vi "Main.vi"(8 "error in (no error)":T2) -> (0 "error out":T2)   [LabVIEW 2019, in "DataManagment.lvlib"]
doc: "Manages burst data\n\nHandles tx bursts \"library\", collects rx bursts for later retrieving.\nManages bursts in memory and on drive"
uses:
  DataManagment.lvlib
  DM group info.ctl
  module data.ctl
  SubVIs/mmWave data_class/mmWave data.lvclass
  DM signal group.ctl
  Intertarget communication/Command + data + response cluster.ctl
  Intertarget communication/Status + response + data cluster.ctl
  module state.ctl
  DM get burst parameters.ctl
  DM get burst by index parameters.ctl
  5bf6cc24-2521-4779-a80f-885c0f377251.vi
  171e3bb6-d49a-4f23-9fbb-f47b30baaa7f.vi
  a598079f-c5bd-4db8-828d-75a2daebc4d7.vi
  ee899b51-2d5d-4f26-9c2b-9d2f7332cf3c.vi
  697aacd5-9936-4587-9d14-828a3325ba78.vi
  6dd8da64-2a06-40fc-b69d-37d6f9184272.vi
  171e3bb6-d49a-4f23-9fbb-f47b30baaa7f.vi/5cbf4985-03a2-482f-aa1d-412015602fcf.vi
  171e3bb6-d49a-4f23-9fbb-f47b30baaa7f.vi/9ddd5499-773d-48fa-be3a-3edd2f81d7af.vi
  a598079f-c5bd-4db8-828d-75a2daebc4d7.vi/43a70c26-45ca-4555-8713-4d640d2761cd.vi
  a598079f-c5bd-4db8-828d-75a2daebc4d7.vi/532e6f42-99be-4d49-9f37-ebc30de797f6.vi
  ee899b51-2d5d-4f26-9c2b-9d2f7332cf3c.vi/279be3f1-d035-438d-8d75-920168a460ff.vi
  ee899b51-2d5d-4f26-9c2b-9d2f7332cf3c.vi/125f3e28-a4cf-4289-b3e7-931c39c491a6.vi
  697aacd5-9936-4587-9d14-828a3325ba78.vi/bc4ebb1e-c054-43e7-8435-a2cc996418b2.vi
  697aacd5-9936-4587-9d14-828a3325ba78.vi/c68d463f-3934-40a4-88c5-9e6f02909ca2.vi
  6dd8da64-2a06-40fc-b69d-37d6f9184272.vi/4dacbd5d-4013-4b6b-9f66-fc6ac213e238.vi
  6dd8da64-2a06-40fc-b69d-37d6f9184272.vi/8eb97bab-6edf-4927-bcd5-73d21db452ab.vi
  <vilib>/Utility/High Resolution Relative Seconds.vi
  DM GV.vi
  SubVIs/Shared/Comm GV.vi
  <vilib>/addons/_JKI.lib/Serialization/JSON/Library/Unflatten From JSON String.vi
  Intertarget communication/CommandResponse communication.lvlib
  SubVIs/Shared/Shared.lvlib
  <vilib>/addons/_JKI.lib/Serialization/JSON/JKI JSON Serialization.lvlib
panel:
  out "group info":T1 {"Memory" format="%#_6pB"; "burst sizes" format="%#_6p"}
  out "oldest":string
  out "newest":string
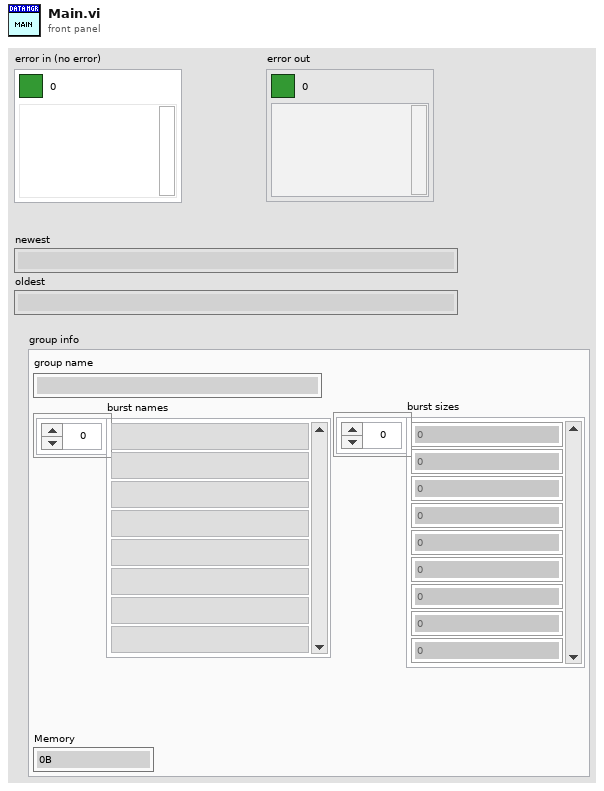
[diagram p1: front panel]
types:
  T1 = typedef "DataManagment.lvlib/DM group info.ctl" = cluster{"group name":string, "burst names":string[], "burst sizes":dbl[], "Memory":dbl}
  T2 = cluster{"Boolean Round":bool, "code":i32, "source":string}
  T3 = typedef "CommandResponse communication.lvlib/Command + data + response cluster.ctl" = cluster{"message":string, "parameters":string, "response notifier":refnum<notifier>, "data":variant}
  T4 = typedef "DataManagment.lvlib/module state.ctl" = enum16{"init", "configure", "run", "close"}
  T5 = typedef "DataManagment.lvlib/module data.ctl" = cluster{"Group names":string[], "Signal groups":map{string, refnum<class "mmWave data.lvclass">}[], "groups":T6[]}
  T6 = typedef "DataManagment.lvlib/DM signal group.ctl" = cluster{"history":string[]}
  T7 = typedef "CommandResponse communication.lvlib/Status + response + data cluster.ctl" = cluster{"message":string, "response":string, "data":variant}
  T8 = typedef "DataManagment.lvlib/DM get burst parameters.ctl" = cluster{"group":string, "bursts":string[]}
  T9 = typedef "DataManagment.lvlib/DM get burst by index parameters.ctl" = cluster{"group":string, "index":i32}
  T10 = map{string, refnum<class "mmWave data.lvclass">}[]
  T11 = cluster{string, refnum<class "mmWave data.lvclass">}
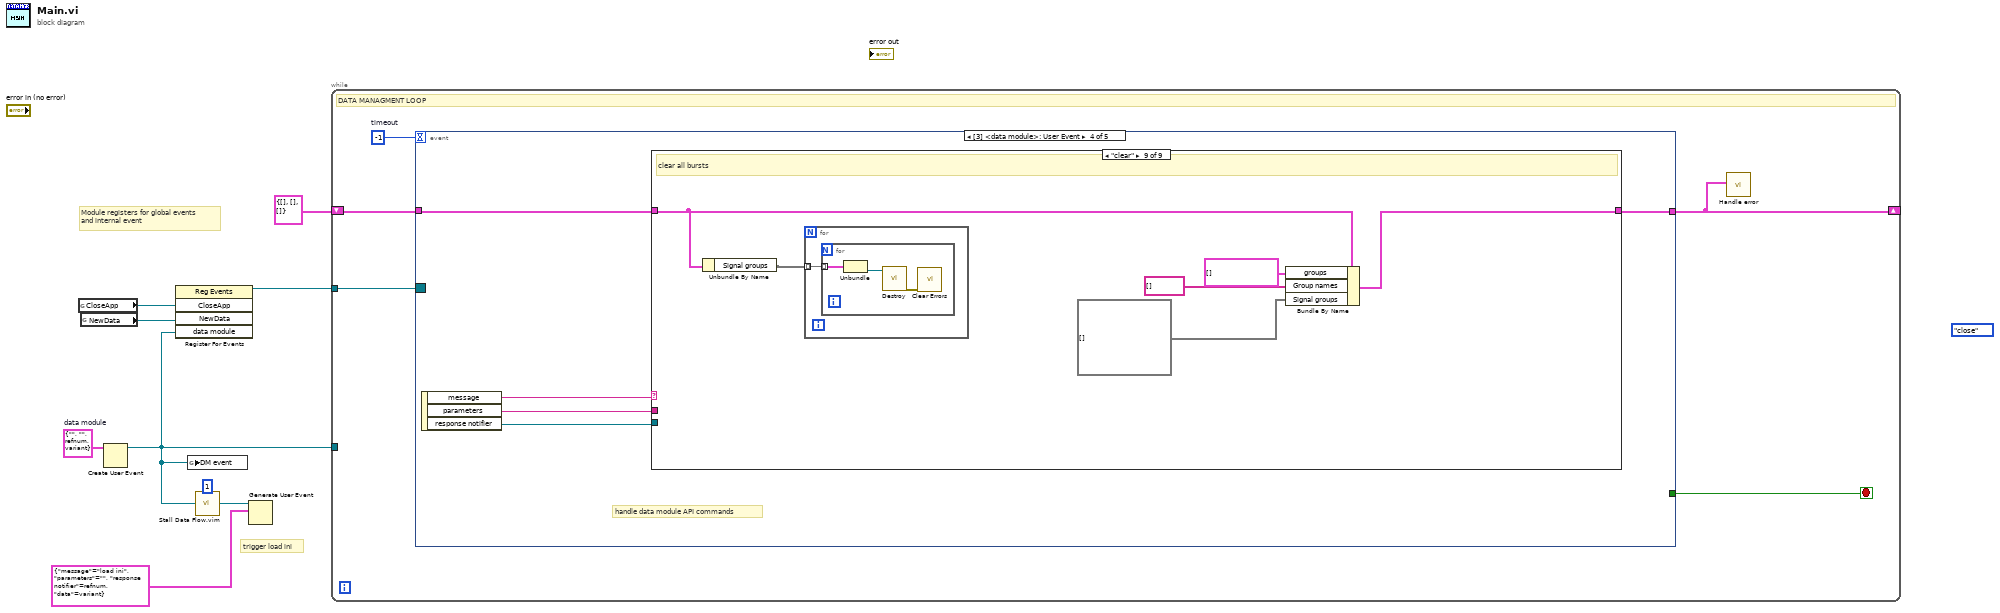
[diagram p0: block diagram]
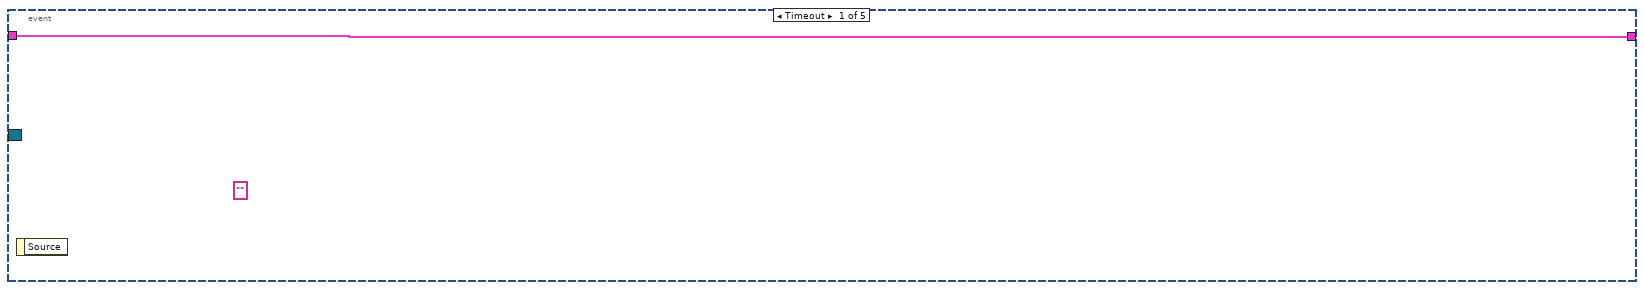
[diagram p2: hidden frame]
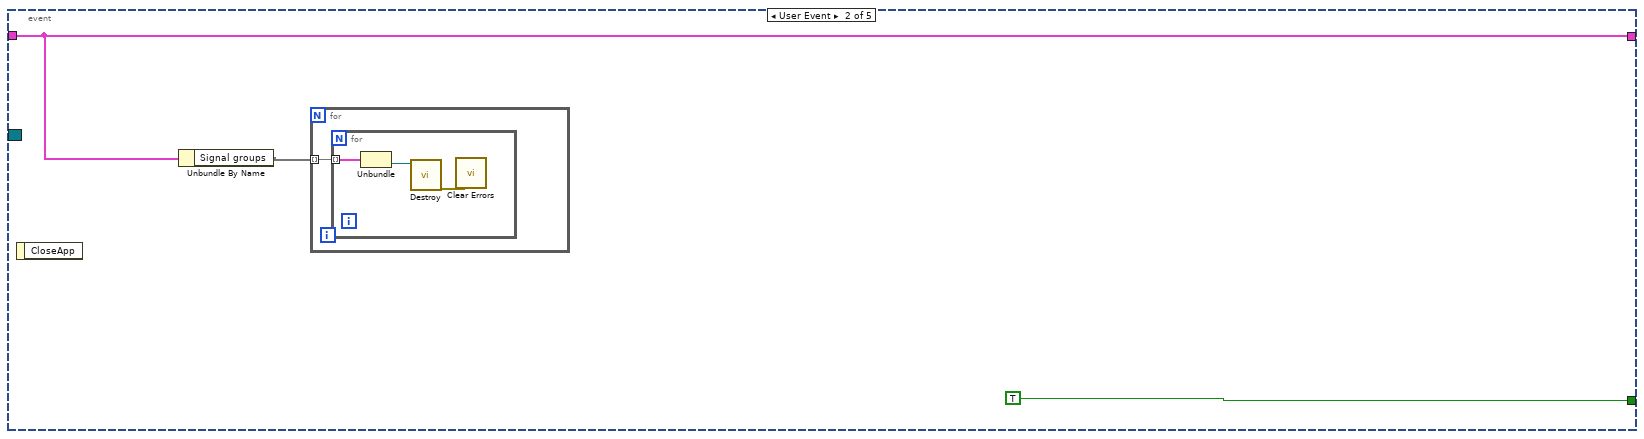
[diagram p3: hidden frame]
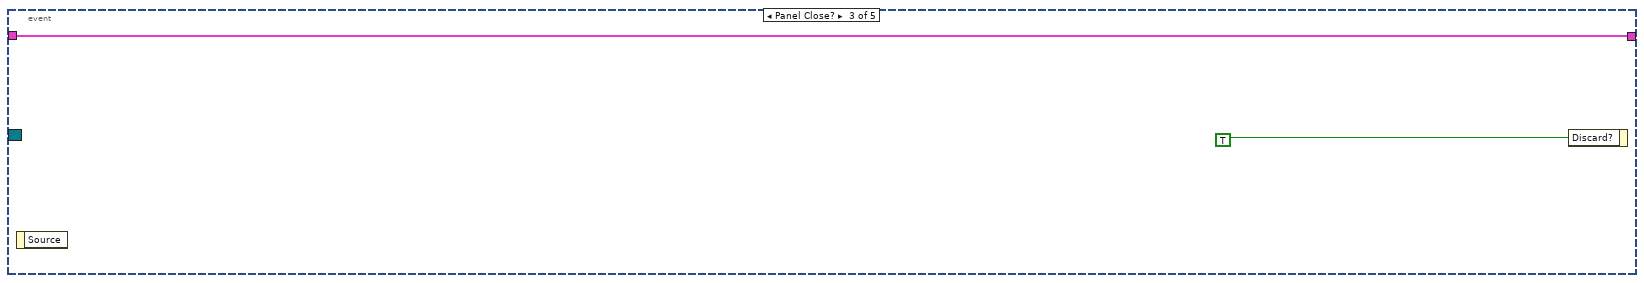
[diagram p4: hidden frame]
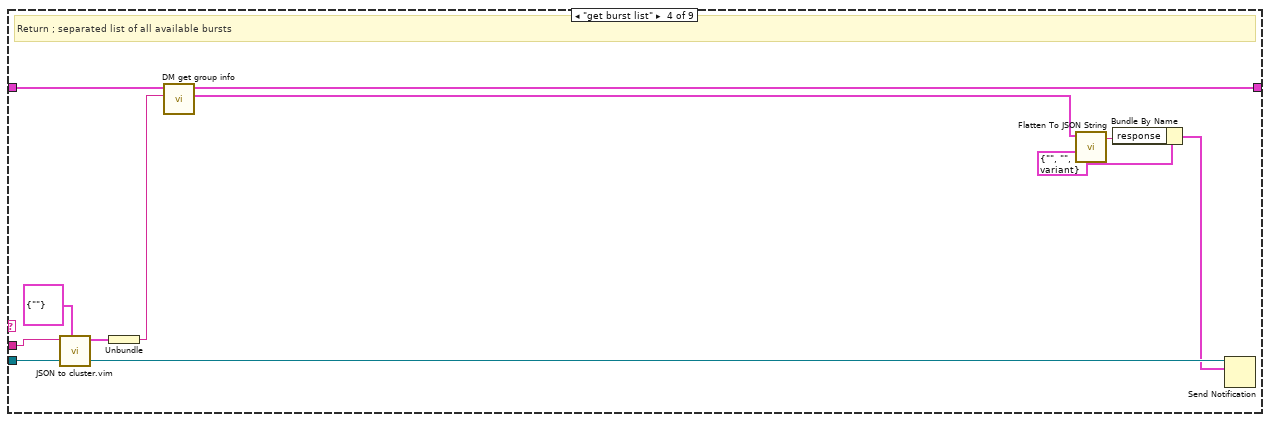
[diagram p8: hidden frame]
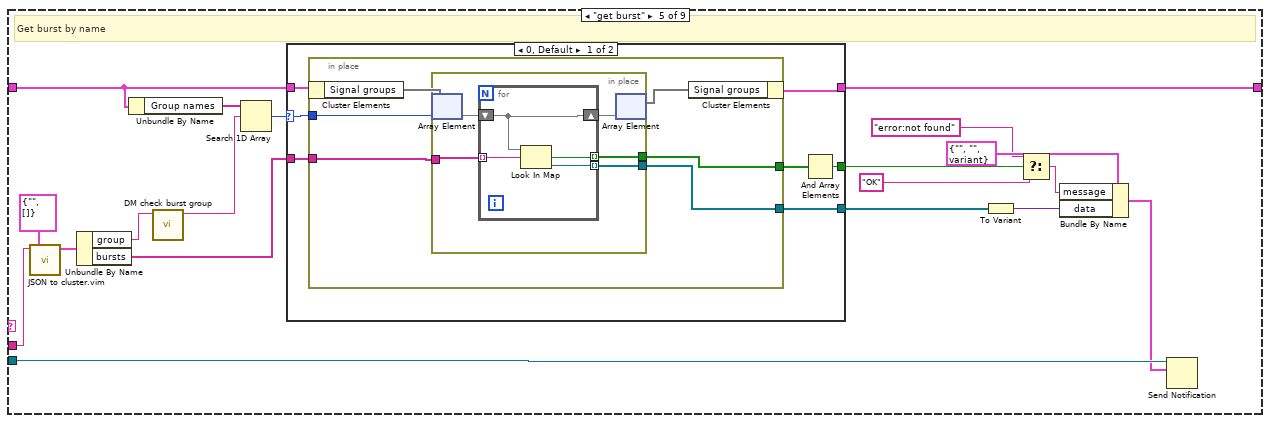
[diagram p9: hidden frame]
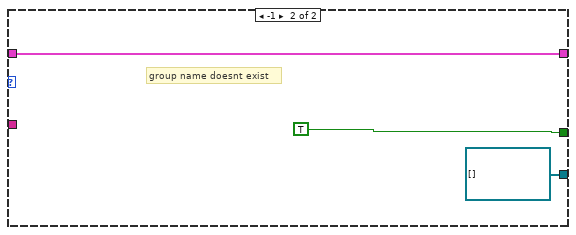
[diagram p10: hidden frame]
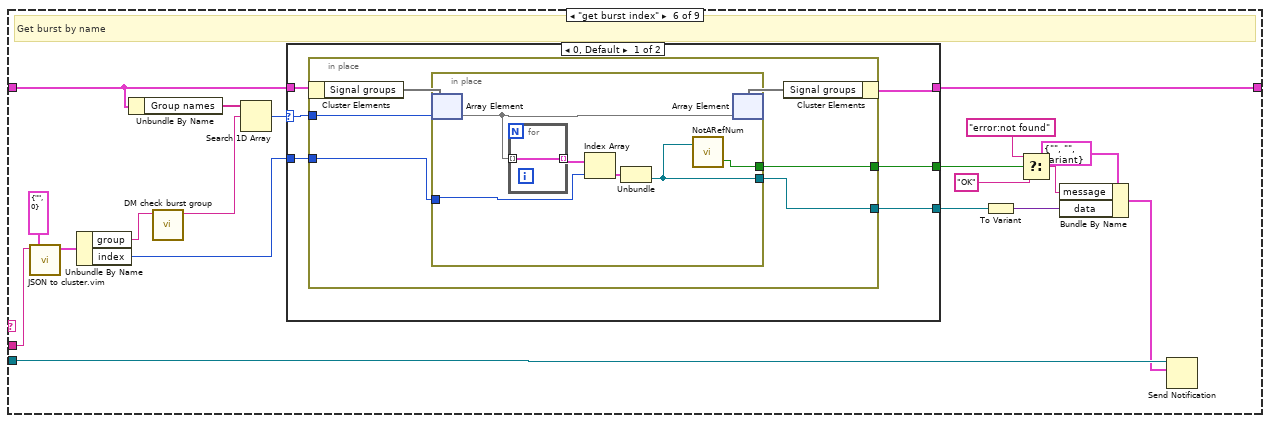
[diagram p11: hidden frame]
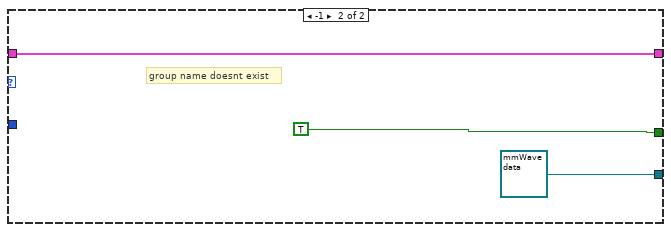
[diagram p12: hidden frame]
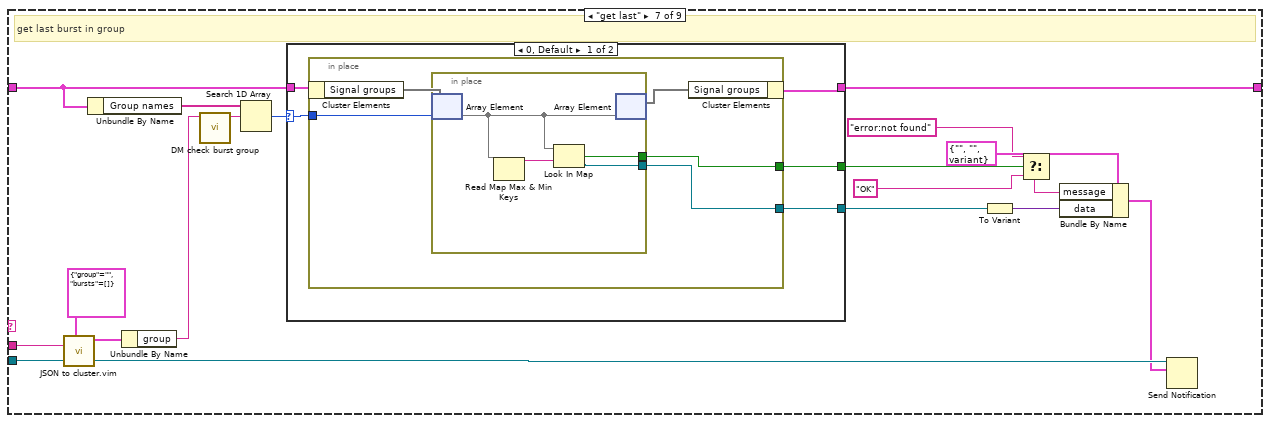
[diagram p13: hidden frame]
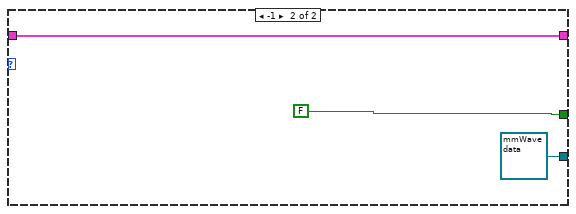
[diagram p14: hidden frame]
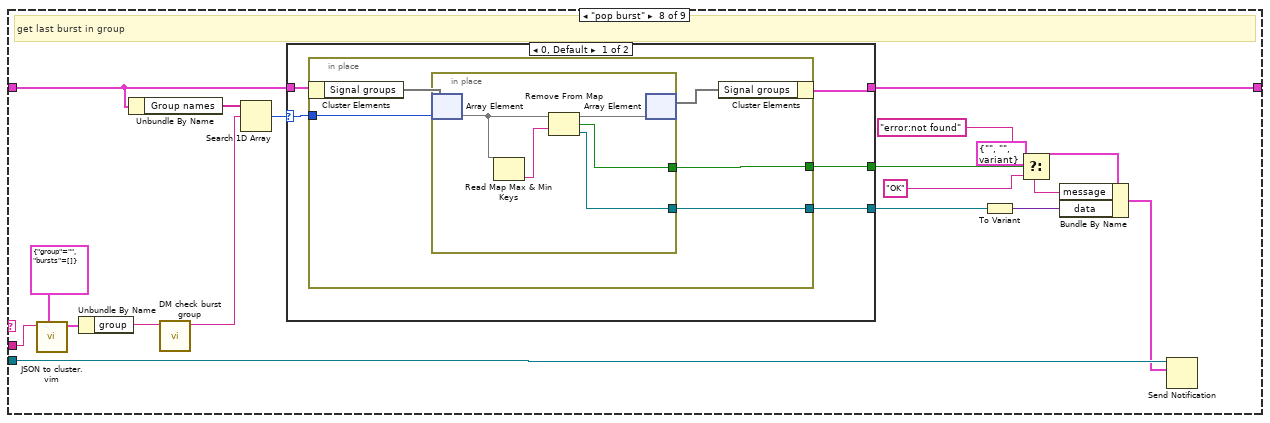
[diagram p15: hidden frame]
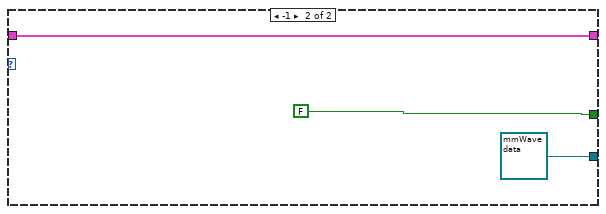
[diagram p16: hidden frame]
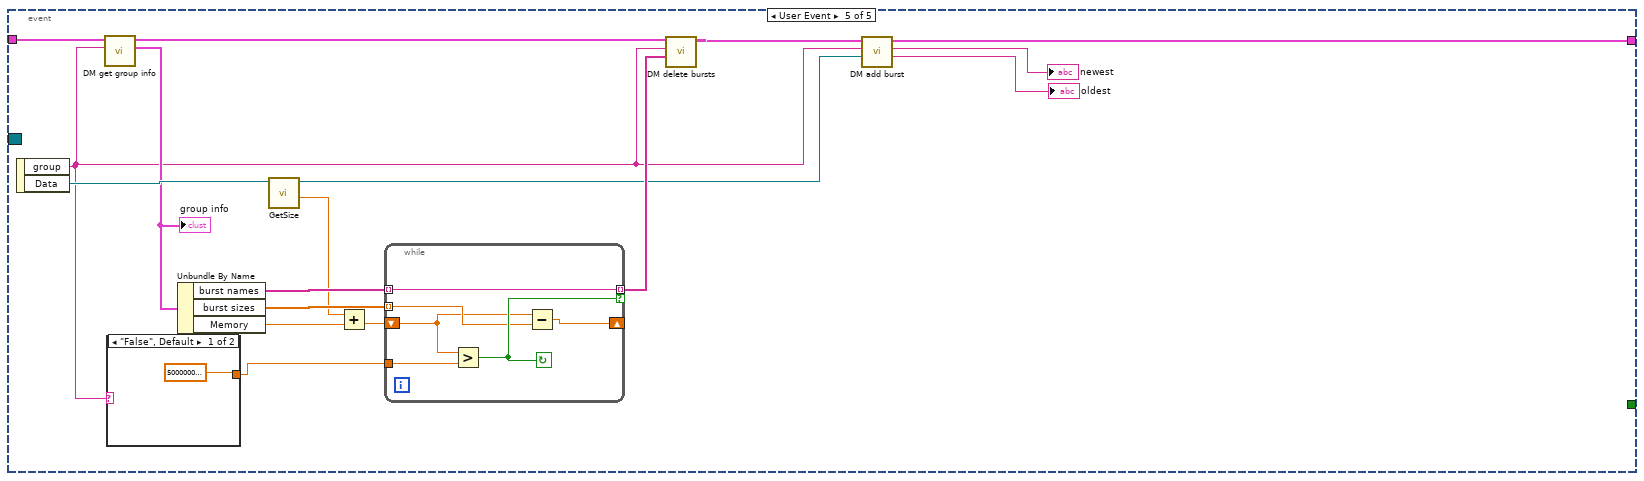
[diagram p17: hidden frame]
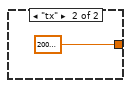
[diagram p18: hidden frame]
diagram:
  w3 = T3 {"message"="", "parameters"="", "response notifier"=refnum, "data"=variant}  # data module
  (unwired) module_state."close" ("module states")
  # "trigger load ini"
  # "Module registers for global events\nand internal event"
  n1 = global read "Comm GV.vi" "CloseApp"() -> (w5:refnum<user-event>)
  n2 = global read "Comm GV.vi" "NewData"() -> (w4:refnum<user-event>)
  n3 = Create User Event(user event datatype=w3) -> (user event=w1:refnum<user-event>)  [unwired: 1 in, 1 out]
  n4 = register-events(w5, w4, w1) -> (reference out=w9:refnum<event-registration>)  [unwired: 2 in, 1 out]
  n5 = global write "DM GV.vi" "DM event"(w1) -> ()
  n6 = call "Stall Data Flow.vim"("value in"=w1, "milliseconds to wait"=u32 1) -> ("value out"=w7:refnum<user-event>)  [unwired: 1 out]
  n7 = Generate User Event(user event=w7, event data cluster=T3 {"message"="load ini", "parameters"="", "response notifier"=refnum, "data"=variant} ("event data")) -> ()  [unwired: 2 in, 2 out]
  n8 = while {
    tunnel: w9 -> [w14]
    tunnel: w1 -> [_]
    shift-right: [w10] -> _
    shift-left: T5 {"Group names"=[], "Signal groups"=[], "groups"=[]} ("module loopdata") -> [w11]
    stop <- w12 stop-if-true
    w13 = -1  # timeout
    # "DATA MANAGMENT LOOP"
    n9 = event shown="[3] <data module>: User Event" {
      selector: w14 -> [_ _ _ _ _]
      dyn-events: _ -> [_ _ _ _ _]
      timeout: w13 -> [_ _ _ _ _]
      tunnel: [_ TRUE _ _ _] -> w12
      tunnel: [w15 w16 w23 w28 w226] -> w10
      tunnel: w11 -> [w15 w16 w23 w29 w223]
      event Timeout {
        (unwired) "" ("message")
        n10 = event-data() -> ()  [unwired: 1 in, 1 out]
      }
      event User Event {
        n11 = event-data() -> ()  [unwired: 1 in, 1 out]
        n12 = Unbundle By Name(w16) -> ("Signal groups"=w17:T10)
        n13 = for {
          tunnel: w17 -> [w19] mode=indexing
          n14 = for {
            tunnel: w19 -> [w22] mode=indexing
            n15 = Unbundle(w22) -> (w21:refnum<class "mmWave data.lvclass">)  [unwired: 1 out]
            n16 = call-dynamic "Destroy.vi"("reference in"=w21) -> ("error out"=w20:errorcluster)  [unwired: 17 in, 1 out]
            n17 = call <vilib>:"Clear Errors.vi"("error in (no error)"=w20) -> ()  [unwired: 5 in, 2 out]
          }
        }
      }
      event Panel Close? {
        n18 = event-data() -> ()  [unwired: 1 in, 1 out]
        n19 = event-data("Discard?"=TRUE) -> ()  [unwired: 1 in, 1 out]
      }
      event User Event {
        # "handle data module API commands"
        n20 = event-data() -> ("message"=w26:string, "parameters"=w25:string, "response notifier"=w27:refnum<notifier>)  [unwired: 1 in]
        n21 = case shown="\"clear\"" w26 {
          tunnel: w29 -> [w30 w31 w32 w43 w51 w95 w135 w170 w204]
          tunnel: [w30 w31 w32 w39 w52 w96 w136 w171 w203] -> w28
          tunnel: w27 -> [_ _ _ w42 w62 w106 w146 w181 _]
          tunnel: w25 -> [_ _ _ w38 w48 w92 w133 w167 _]
          frame Default {
          }
          frame "load ini" {
          }
          frame "---DATA HANDLING---" {
          }
          frame "get burst list" {
            # "Return ; separated list of all available bursts"
            n22 = call "JSON to cluster.vim"("data"=cluster{"group":string} {"group"=""}, "JSON in"=w38) -> ("data"=w36:cluster{"group":string})  [unwired: 7 in, 2 out]
            n23 = Unbundle(w36) -> ("group"=w33:string)
            n24 = call "DM get group info.vi"("group"=w33, "module loopdata in"=w43) -> ("group info"=w34:T1, "module loopdata out"=w39:T5)  [unwired: 8 in]
            n25 = call <vilib>:"Flatten To JSON String.vi"("Variant"=w34) -> ("JSON String"=w35:string)  [unwired: 9 in, 1 out]
            n26 = Bundle By Name(cluster=T7 {"message"="", "response"="", "data"=variant} ("notification"), "response"=w35) -> (w40:T7)
            n27 = Send Notification(notification=w40, notifier=w42) -> ()  [unwired: 1 in, 2 out]
          }
          frame "get burst" {
            # "Get burst by name"
            n28 = call "JSON to cluster.vim"("data"=T8 {"group"="", "bursts"=[]} ("Cluster"), "JSON in"=w48) -> ("data"=w46:T8)  [unwired: 7 in, 2 out]
            n29 = Unbundle By Name(w46) -> ("group"=w45:string, "bursts"=w50:string[])
            n30 = Unbundle By Name(w51) -> ("Group names"=w55:string[])
            n31 = call "DM check burst group.vi"("group"=w45) -> ("String"=w44:string)  [unwired: 10 in]
            n32 = Search 1D Array(1D array=w55, element=w44) -> (index of element=w54:i32)  [unwired: 1 in]
            n33 = case shown="0, Default" w54 {
              selector: w54 -> [w66 _]
              tunnel: [w69 TRUE] -> w53
              tunnel: [w67 w86] -> w52
              tunnel: w51 -> [w68 w86]
              tunnel: w50 -> [w65 _]
              tunnel: [w64 refnum<class "mmWave data.lvclass">[] []] -> w49
              frame 0, Default {
                n34 = in-place {
                  in-place-border: w66 -> [w73]
                  in-place-border: w65 -> [w72]
                  in-place-border: [w71] -> w64
                  in-place-border: [w70] -> w63
                  n35 = in-place-cluster #1(w68) -> ("Signal groups"=w75:T10)
                  n36 = in-place {
                    in-place-border: w72 -> [w78]
                    in-place-border: [w77] -> w71
                    in-place-border: [w76] -> w70
                    n37 = in-place-array #2(w75, w73) -> (w80:map{string, refnum<class "mmWave data.lvclass">})
                    n38 = for {
                      shift-right: [w84] -> w79
                      shift-left: w80 -> [w84]
                      tunnel: w78 -> [w83] mode=indexing
                      tunnel: [w82] -> w77 mode=indexing
                      tunnel: [w81] -> w76 mode=indexing
                      n39 = Look In Map(map=w84, key=w83) -> (key not found?=w81:bool, value=w82:refnum<class "mmWave data.lvclass">)  [unwired: 1 in]
                    }
                    n40 = in-place-array #2(w79) -> (w74:T10)  [unwired: 1 out]
                  }
                  n41 = in-place-cluster #1("Signal groups"=w74) -> (w67:T5)
                }
                n42 = And Array Elements(Boolean array=w63) -> (logical AND=w69:bool)
              }
              frame -1 {
                # "group name doesnt exist"
              }
            }
            n43 = To Variant(anything=w49) -> (Variant=w59:variant)
            n44 = Select(t="error:not found", s=w53, f="OK") -> (s? t:f=w56:string)
            n45 = Bundle By Name(cluster=T7 {"message"="", "response"="", "data"=variant} ("notification"), "message"=w56, "data"=w59) -> (w60:T7)
            n46 = Send Notification(notification=w60, notifier=w62) -> ()  [unwired: 1 in, 2 out]
          }
          frame "get burst index" {
            # "Get burst by name"
            n47 = call "JSON to cluster.vim"("data"=T9 {"group"="", "index"=0} ("Cluster"), "JSON in"=w92) -> ("data"=w90:T9)  [unwired: 7 in, 2 out]
            n48 = Unbundle By Name(w90) -> ("group"=w89:string, "index"=w94:i32)
            n49 = Unbundle By Name(w95) -> ("Group names"=w99:string[])
            n50 = call "DM check burst group.vi"("group"=w89) -> ("String"=w88:string)  [unwired: 10 in]
            n51 = Search 1D Array(1D array=w99, element=w88) -> (index of element=w98:i32)  [unwired: 1 in]
            n52 = case shown="0, Default" w98 {
              selector: w98 -> [w110 _]
              tunnel: [w107 TRUE] -> w97
              tunnel: [w111 w127] -> w96
              tunnel: w95 -> [w112 w127]
              tunnel: w94 -> [w109 _]
              tunnel: [w108 refnum<class "mmWave data.lvclass"> refnum] -> w93
              frame 0, Default {
                n53 = in-place {
                  in-place-border: w110 -> [w116]
                  in-place-border: w109 -> [w115]
                  in-place-border: [w114] -> w108
                  in-place-border: [w113] -> w107
                  n54 = in-place-cluster #3(w112) -> ("Signal groups"=w118:T10)
                  n55 = in-place {
                    in-place-border: w115 -> [w123]
                    in-place-border: [w120] -> w114
                    in-place-border: [w119] -> w113
                    n56 = in-place-array #4(w118, w116) -> (w124:map{string, refnum<class "mmWave data.lvclass">})
                    n57 = for {
                      tunnel: w124 -> [w125] mode=indexing
                      tunnel: [w125] -> w122 mode=indexing
                    }
                    n58 = Index Array(array=w122, index=w123) -> (element=w121:T11)
                    n59 = Unbundle(w121) -> (w120:refnum<class "mmWave data.lvclass">)  [unwired: 1 out]
                    n60 = call-dynamic "NotARefNum.vi"("reference in"=w120) -> ("not a refnum?"=w119:bool)  [unwired: 1 in, 1 out]
                    n61 = in-place-array #4(w124) -> (w117:T10)  [unwired: 1 out]
                  }
                  n62 = in-place-cluster #3("Signal groups"=w117) -> (w111:T5)
                }
              }
              frame -1 {
                # "group name doesnt exist"
              }
            }
            n63 = To Variant(anything=w93) -> (Variant=w103:variant)
            n64 = Select(t="error:not found", s=w97, f="OK") -> (s? t:f=w100:string)
            n65 = Bundle By Name(cluster=T7 {"message"="", "response"="", "data"=variant} ("notification"), "message"=w100, "data"=w103) -> (w104:T7)
            n66 = Send Notification(notification=w104, notifier=w106) -> ()  [unwired: 1 in, 2 out]
          }
          frame "get last" {
            # "get last burst in group"
            n67 = call "JSON to cluster.vim"("data"=T8 {"group"="", "bursts"=[]} ("Cluster"), "JSON in"=w133) -> ("data"=w131:T8)  [unwired: 7 in, 2 out]
            n68 = Unbundle By Name(w135) -> ("Group names"=w139:string[])
            n69 = Unbundle By Name(w131) -> ("group"=w130:string)
            n70 = call "DM check burst group.vi"("group"=w130) -> ("String"=w129:string)  [unwired: 10 in]
            n71 = Search 1D Array(1D array=w139, element=w129) -> (index of element=w138:i32)  [unwired: 1 in]
            n72 = case shown="0, Default" w138 {
              selector: w138 -> [w149 _]
              tunnel: [w148 FALSE] -> w137
              tunnel: [w150 w162] -> w136
              tunnel: w135 -> [w151 w162]
              tunnel: [w147 refnum<class "mmWave data.lvclass"> refnum] -> w134
              frame 0, Default {
                n73 = in-place {
                  in-place-border: w149 -> [w154]
                  in-place-border: [w153] -> w147
                  in-place-border: [w152] -> w148
                  n74 = in-place-cluster #5(w151) -> ("Signal groups"=w156:T10)
                  n75 = in-place {
                    in-place-border: [w159] -> w153
                    in-place-border: [w158] -> w152
                    n76 = in-place-array #6(w156, w154) -> (w157:map{string, refnum<class "mmWave data.lvclass">})
                    n77 = Read Map Max & Min Keys(11:w157) -> (3:w160:string)  [unwired: 1 out]
                    n78 = Look In Map(map=w157, key=w160) -> (key not found?=w158:bool, value=w159:refnum<class "mmWave data.lvclass">)  [unwired: 1 in]
                    n79 = in-place-array #6(w157) -> (w155:T10)  [unwired: 1 out]
                  }
                  n80 = in-place-cluster #5("Signal groups"=w155) -> (w150:T5)
                }
              }
              frame -1 {
              }
            }
            n81 = To Variant(anything=w134) -> (Variant=w143:variant)
            n82 = Select(t="error:not found", s=w137, f="OK") -> (s? t:f=w140:string)
            n83 = Bundle By Name(cluster=T7 {"message"="", "response"="", "data"=variant} ("notification"), "message"=w140, "data"=w143) -> (w144:T7)
            n84 = Send Notification(notification=w144, notifier=w146) -> ()  [unwired: 1 in, 2 out]
          }
          frame "pop burst" {
            # "get last burst in group"
            n85 = call "JSON to cluster.vim"("data"=T8 {"group"="", "bursts"=[]} ("Cluster"), "JSON in"=w167) -> ("data"=w166:T8)  [unwired: 7 in, 2 out]
            n86 = Unbundle By Name(w166) -> ("group"=w165:string)
            n87 = Unbundle By Name(w170) -> ("Group names"=w174:string[])
            n88 = call "DM check burst group.vi"("group"=w165) -> ("String"=w164:string)  [unwired: 10 in]
            n89 = Search 1D Array(1D array=w174, element=w164) -> (index of element=w173:i32)  [unwired: 1 in]
            n90 = case shown="0, Default" w173 {
              selector: w173 -> [w184 _]
              tunnel: [w183 FALSE] -> w172
              tunnel: [w185 w198] -> w171
              tunnel: w170 -> [w186 w198]
              tunnel: [w182 refnum<class "mmWave data.lvclass"> refnum] -> w169
              frame 0, Default {
                n91 = in-place {
                  in-place-border: w184 -> [w189]
                  in-place-border: [w188] -> w182
                  in-place-border: [w187] -> w183
                  n92 = in-place-cluster #7(w186) -> ("Signal groups"=w191:T10)
                  n93 = in-place {
                    in-place-border: [w193] -> w188
                    in-place-border: [w192] -> w187
                    n94 = in-place-array #8(w191, w189) -> (w196:map{string, refnum<class "mmWave data.lvclass">})
                    n95 = Read Map Max & Min Keys(11:w196) -> (1:w195:string)  [unwired: 1 out]
                    n96 = Remove From Map(10:w195, 11:w196) -> (1:w193:refnum<class "mmWave data.lvclass">, 2:w192:bool, 3:w194:map{string, refnum<class "mmWave data.lvclass">})
                    n97 = in-place-array #8(w194) -> (w190:T10)  [unwired: 1 out]
                  }
                  n98 = in-place-cluster #7("Signal groups"=w190) -> (w185:T5)
                }
              }
              frame -1 {
              }
            }
            n99 = To Variant(anything=w169) -> (Variant=w178:variant)
            n100 = Select(t="error:not found", s=w172, f="OK") -> (s? t:f=w175:string)
            n101 = Bundle By Name(cluster=T7 {"message"="", "response"="", "data"=variant} ("notification"), "message"=w175, "data"=w178) -> (w179:T7)
            n102 = Send Notification(notification=w179, notifier=w181) -> ()  [unwired: 1 in, 2 out]
          }
          frame "clear" {
            # "clear all bursts"
            n103 = Unbundle By Name(w204) -> ("Signal groups"=w205:T10)
            n104 = for {
              tunnel: w205 -> [w206] mode=indexing
              n105 = for {
                tunnel: w206 -> [w209] mode=indexing
                n106 = Unbundle(w209) -> (w208:refnum<class "mmWave data.lvclass">)  [unwired: 1 out]
                n107 = call-dynamic "Destroy.vi"("reference in"=w208) -> ("error out"=w207:errorcluster)  [unwired: 17 in, 1 out]
                n108 = call <vilib>:"Clear Errors.vi"("error in (no error)"=w207) -> ()  [unwired: 5 in, 2 out]
              }
            }
            n109 = Bundle By Name(cluster=w204, "groups"=T6[] [], "Group names"=string[] [], "Signal groups"=T10 []) -> (w203:T5)
          }
        }
      }
      event User Event {
        n110 = event-data() -> ("group"=w210:string, "Data"=w222:refnum<class "mmWave data.lvclass">)  [unwired: 1 in]
        n111 = call "DM get group info.vi"("group"=w210, "module loopdata in"=w223) -> ("group info"=w221:T1, "module loopdata out"=w216:T5)  [unwired: 8 in]
        "group info" <- w221
        n112 = case shown="\"False\", Default" w210 {
          tunnel: [500000000.0 ("max size") 2000000000.0 ("max size")] -> w217
          frame "False", Default {
          }
          frame "tx" {
          }
        }
        n113 = Unbundle By Name(w221) -> ("burst names"=w220:string[], "burst sizes"=w219:dbl[], "Memory"=w218:dbl)
        n114 = call-dynamic "GetSize.vi"("reference in"=w222) -> ("Size (Bytes)"=w211:dbl, "reference out"=w213:refnum<class "mmWave data.lvclass">)  [unwired: 7 in, 2 out]
        n115 = Add(x=w211, y=w218) -> (x+y=w212:dbl)
        n116 = while {
          shift-right: [w229] -> _
          shift-left: w212 -> [w230]
          tunnel: w217 -> [w234]
          tunnel: w220 -> [w233] mode=indexing
          tunnel: w219 -> [w231] mode=indexing
          tunnel: [w233] -> w215 mode=indexing if=w232
          stop <- w232 continue-if-true
          n117 = Greater?(x=w230, y=w234) -> (0:w232:bool)
          n118 = Subtract(x=w230, y=w231) -> (x-y=w229:dbl)
        }
        n119 = call "DM delete bursts.vi"("bursts to delete"=w215, "group"=w210, "module loopdata in"=w216) -> ("module loopdata out"=w214:T5)  [unwired: 8 in]
        n120 = call "DM add burst.vi"("mmWave data in"=w213, "group"=w210, "module loopdata in"=w214) -> ("oldest"=→"oldest":string, "newest"=→"newest":string, "module loopdata out"=w226:T5)  [unwired: 6 in]
      }
    }
    n121 = call "Handle error.vi"("module loopdata"=w10) -> ()  [unwired: 11 in]
  }
